vi "Close Dialog.vi"(5 "error in (no error)":errorcluster, 8 "Only in RTE (T)":bool=TRUE) -> (0 "error out":errorcluster)   [LabVIEW 2013]
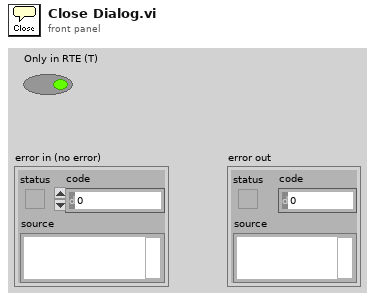
[diagram p1: front panel]
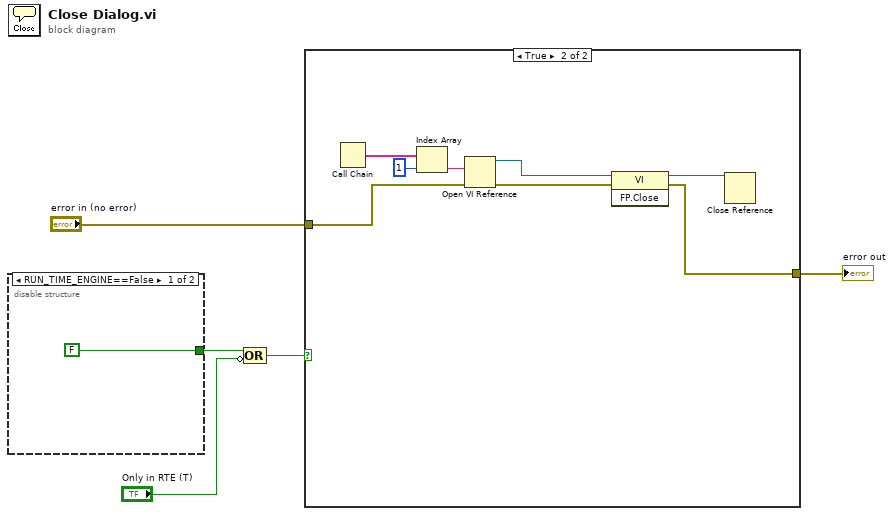
[diagram p0: block diagram]
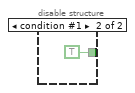
[diagram p3: hidden frame]
diagram:
  n1 = disable-structure shown="RUN_TIME_ENGINE==False" {
    disable-tunnel: [FALSE ("exe-file?") TRUE ("exe-file?")] -> w3
    frame condition #0 (active) {
    }
    frame condition #1 {
    }
  }
  n2 = Compound Arithmetic op=OR(w3, invert "Only in RTE (T)") -> (w1:bool)
  n3 = case shown="True" w1 {
    tunnel: "error in (no error)" -> [w8 w13]
    tunnel: [w8 w12] -> w4
    frame False {
    }
    frame True {
      n4 = Call Chain() -> (call chain=w16:string[])
      n5 = Index Array(array=w16, index=1) -> (element=w14:string)
      n6 = Open VI Reference(vi path=w14, error in (no error)=w13) -> (vi reference=w11:refnum<vi>, error out=w10:errorcluster)  [unwired: 4 out]
      n7 = invoke class="VI" method="FP.Close"(reference=w11, error in=w10) -> (reference out=w9:refnum<vi>, error out=w12:errorcluster)  [unwired: 1 in, 1 out]
      n8 = Close Reference(reference=w9) -> ()  [unwired: 1 in, 1 out]
    }
  }
  "error out" <- w4
